vi "Main.vi"(11 "Module Admin":refnum<class "Delacor_lib_QMH_Module Admin.lvclass">) -> ()   [LabVIEW 2023, in "Dispatcher.lvlib"]
doc: "This template is based off of the Queued Message Handler design pattern and the Queued Message Handler project template that ships with LabVIEW.\n\nThe main difference is that the queue is private to this module and communication between modules is performed via Broadcast and Request events.\n\nRequest events are wrapped in public API methods and are handled in the Event Handling Loop (EHL) of this VI. Any module can register for Broadcast events sent by this module. The EHL generates messages based on user interface actions.\n\nThe Message Handling Loop (MHL) processes messages generated by the EHL, or by other messages. The messages are string values, so new messages can be added easily to the Message Cases case structure in the MHL. Each message cluster can also provide an optional value for Message Data, which is a variant that can be converted to whatever message-specific data is required.\n_____\nBased on DQMH Project Template 6.1.0.94."
uses:
  Dispatcher.lvlib
  <vilib>/Delacor/Delacor QMH/Libraries/Message Queue_class/Delacor_lib_QMH_Message Queue.lvclass
  Module Data--cluster.ctl
  <vilib>/Utility/miscctls.llb/LVPointTypeDef.ctl
  <vilib>/Utility/error.llb/Error Cluster From Error Code.vi
  <vilib>/ErrorRing/Error Ring.xnode
  <vilib>/Delacor/Delacor QMH/Libraries/Message Queue_class/Delacor_lib_QMH_Enqueue Message (Single).vi
  Stop Argument--cluster.ctl
  <vilib>/Delacor/Delacor QMH/Libraries/Module Admin_class/Delacor_lib_QMH_Module Admin.lvclass
  Registration/Registration.lvlib
  Graph_data_collector/Graph_data_collector.lvlib
  Initial Data/Initial Data.lvlib
  Registration/Data_reg.ctl
  Graph_data_collector/Data Control.ctl
  <vilib>/Delacor/Delacor QMH/Libraries/Message Queue_class/Delacor_lib_QMH_Enqueue Message (Array).vi
panel:
  out "error out":errorcluster
  # "Загрузка......"
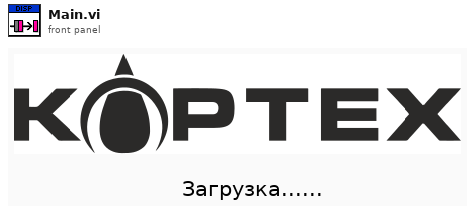
[diagram p1: front panel]
types:
  T1 = typedef "Dispatcher.lvlib/Request Events--cluster.ctl" = cluster{"Stop Module":refnum<user-event>, "Show Panel":refnum<user-event>, "Hide Panel":refnum<user-event>, "Get Module Execution Status":refnum<user-event>, "Show Diagram":refnum<user-event>}
  T2 = typedef "Calculator.lvlib/Broadcast Events--cluster.ctl" = cluster{"Module Did Init":refnum<user-event>, "Status Updated":refnum<user-event>, "Error Reported":refnum<user-event>, "Module Did Stop":refnum<user-event>, "Update Module Execution Status":refnum<user-event>}
  T3 = typedef "Pressure Control System.lvlib/Broadcast Events--cluster.ctl" = cluster{"Module Did Init":refnum<user-event>, "Status Updated":refnum<user-event>, "Error Reported":refnum<user-event>, "Module Did Stop":refnum<user-event>, "Update Module Execution Status":refnum<user-event>}
  T4 = typedef "Automatic.lvlib/Broadcast Events--cluster.ctl" = cluster{"Module Did Init":refnum<user-event>, "Status Updated":refnum<user-event>, "Error Reported":refnum<user-event>, "Module Did Stop":refnum<user-event>, "Update Module Execution Status":refnum<user-event>, "Next Step":refnum<user-event>}
  T5 = typedef "Heat UI.lvlib/Broadcast Events--cluster.ctl" = cluster{"Module Did Init":refnum<user-event>, "Status Updated":refnum<user-event>, "Error Reported":refnum<user-event>, "Module Did Stop":refnum<user-event>, "Update Module Execution Status":refnum<user-event>, "T Data":refnum<user-event>}
  T6 = typedef "DMX.lvlib/Broadcast Events--cluster.ctl" = cluster{"Module Did Init":refnum<user-event>, "Status Updated":refnum<user-event>, "Error Reported":refnum<user-event>, "Module Did Stop":refnum<user-event>, "Update Module Execution Status":refnum<user-event>, "DMX Data":refnum<user-event>}
  T7 = typedef "Initial Data.lvlib/Broadcast Events--cluster.ctl" = cluster{"Module Did Init":refnum<user-event>, "Status Updated":refnum<user-event>, "Error Reported":refnum<user-event>, "Module Did Stop":refnum<user-event>, "Update Module Execution Status":refnum<user-event>, "Data":refnum<user-event>}
  T8 = typedef "LCR GWinstek.lvlib/Broadcast Events--cluster.ctl" = cluster{"Module Did Init":refnum<user-event>, "Status Updated":refnum<user-event>, "Error Reported":refnum<user-event>, "Module Did Stop":refnum<user-event>, "Update Module Execution Status":refnum<user-event>, "LCR Data":refnum<user-event>}
  T9 = typedef "Manual.lvlib/Broadcast Events--cluster.ctl" = cluster{"Module Did Init":refnum<user-event>, "Status Updated":refnum<user-event>, "Error Reported":refnum<user-event>, "Module Did Stop":refnum<user-event>, "Update Module Execution Status":refnum<user-event>, "Pump Data":refnum<user-event>}
  T10 = typedef "Separator UZ.lvlib/Broadcast Events--cluster.ctl" = cluster{"Module Did Init":refnum<user-event>, "Status Updated":refnum<user-event>, "Error Reported":refnum<user-event>, "Module Did Stop":refnum<user-event>, "Update Module Execution Status":refnum<user-event>, "Time Data":refnum<user-event>}
  T11 = typedef "Graph_data_collector.lvlib/Broadcast Events--cluster.ctl" = cluster{"Module Did Init":refnum<user-event>, "Status Updated":refnum<user-event>, "Error Reported":refnum<user-event>, "Module Did Stop":refnum<user-event>, "Update Module Execution Status":refnum<user-event>}
  T12 = typedef "Registration.lvlib/Broadcast Events--cluster.ctl" = cluster{"Module Did Init":refnum<user-event>, "Status Updated":refnum<user-event>, "Error Reported":refnum<user-event>, "Module Did Stop":refnum<user-event>, "Update Module Execution Status":refnum<user-event>, "Data from Registration":refnum<user-event>, "Get Main VI Reference":refnum<user-event>}
  T13 = typedef "Log Module.lvlib/Broadcast Events--cluster.ctl" = cluster{"Module Did Init":refnum<user-event>, "Status Updated":refnum<user-event>, "Error Reported":refnum<user-event>, "Module Did Stop":refnum<user-event>, "Update Module Execution Status":refnum<user-event>}
  T14 = typedef "Menu.lvlib/Broadcast Events--cluster.ctl" = cluster{"Module Did Init":refnum<user-event>, "Status Updated":refnum<user-event>, "Error Reported":refnum<user-event>, "Module Did Stop":refnum<user-event>, "Update Module Execution Status":refnum<user-event>}
  T15 = typedef "Dispatcher.lvlib/Module Data--cluster.ctl" = cluster{"Status":string, "Data reg":T16}
  T16 = typedef "Registration.lvlib/Data_reg.ctl" = cluster{"Дата":string, "Время":string, "Рпл1, МПа":dbl, "Vпл, см3":dbl, "Рпл2, МПа":dbl, "Ргор, МПа":dbl, "Рэфф, МПа":dbl, "R, Ом":dbl, "dL, мм":dbl, "Ткд, градС":dbl, "Тпрод, мкс":dbl, "Тпоп.1, мкс":dbl, "Тпоп.2, мкс":dbl, "Рдм, МПа":dbl, "Q, мл":dbl, "Тнагр, градС":dbl, "ЦАП, градС":dbl}
  T17 = enum32{"invalid lock state", "Not Locked", "Locked (No Password)", "Password-protected"}
  T18 = typedef "Dispatcher.lvlib/Stop Argument--cluster.ctl" = cluster{"Origin":string, "Exit via Stop Module Req?":bool, "Wait for Module to stop?":bool}
  T19 = typedef "LVPointTypeDef.ctl" = cluster{"Horizontal":i16, "Vertical":i16}
  T20 = enum32{"Invalid", "Standard", "Closed", "Hidden", "Minimized", "Maximized"}
  T21 = typedef "Graph_data_collector.lvlib/Data Control.ctl" = cluster{"Время":dbl, "Рпл1, МПа":dbl, "Vпл, см3":dbl, "Рпл2, МПа":dbl, "Ргор, МПа":dbl, "Ткд, градС":dbl, "R, Ом":dbl, "dL, мм":dbl, "Рэфф, МПа":dbl, "Рдм, МПа":dbl, "Q, мл":dbl, "Тнагр, градС":dbl, "ЦАП, градС":dbl}
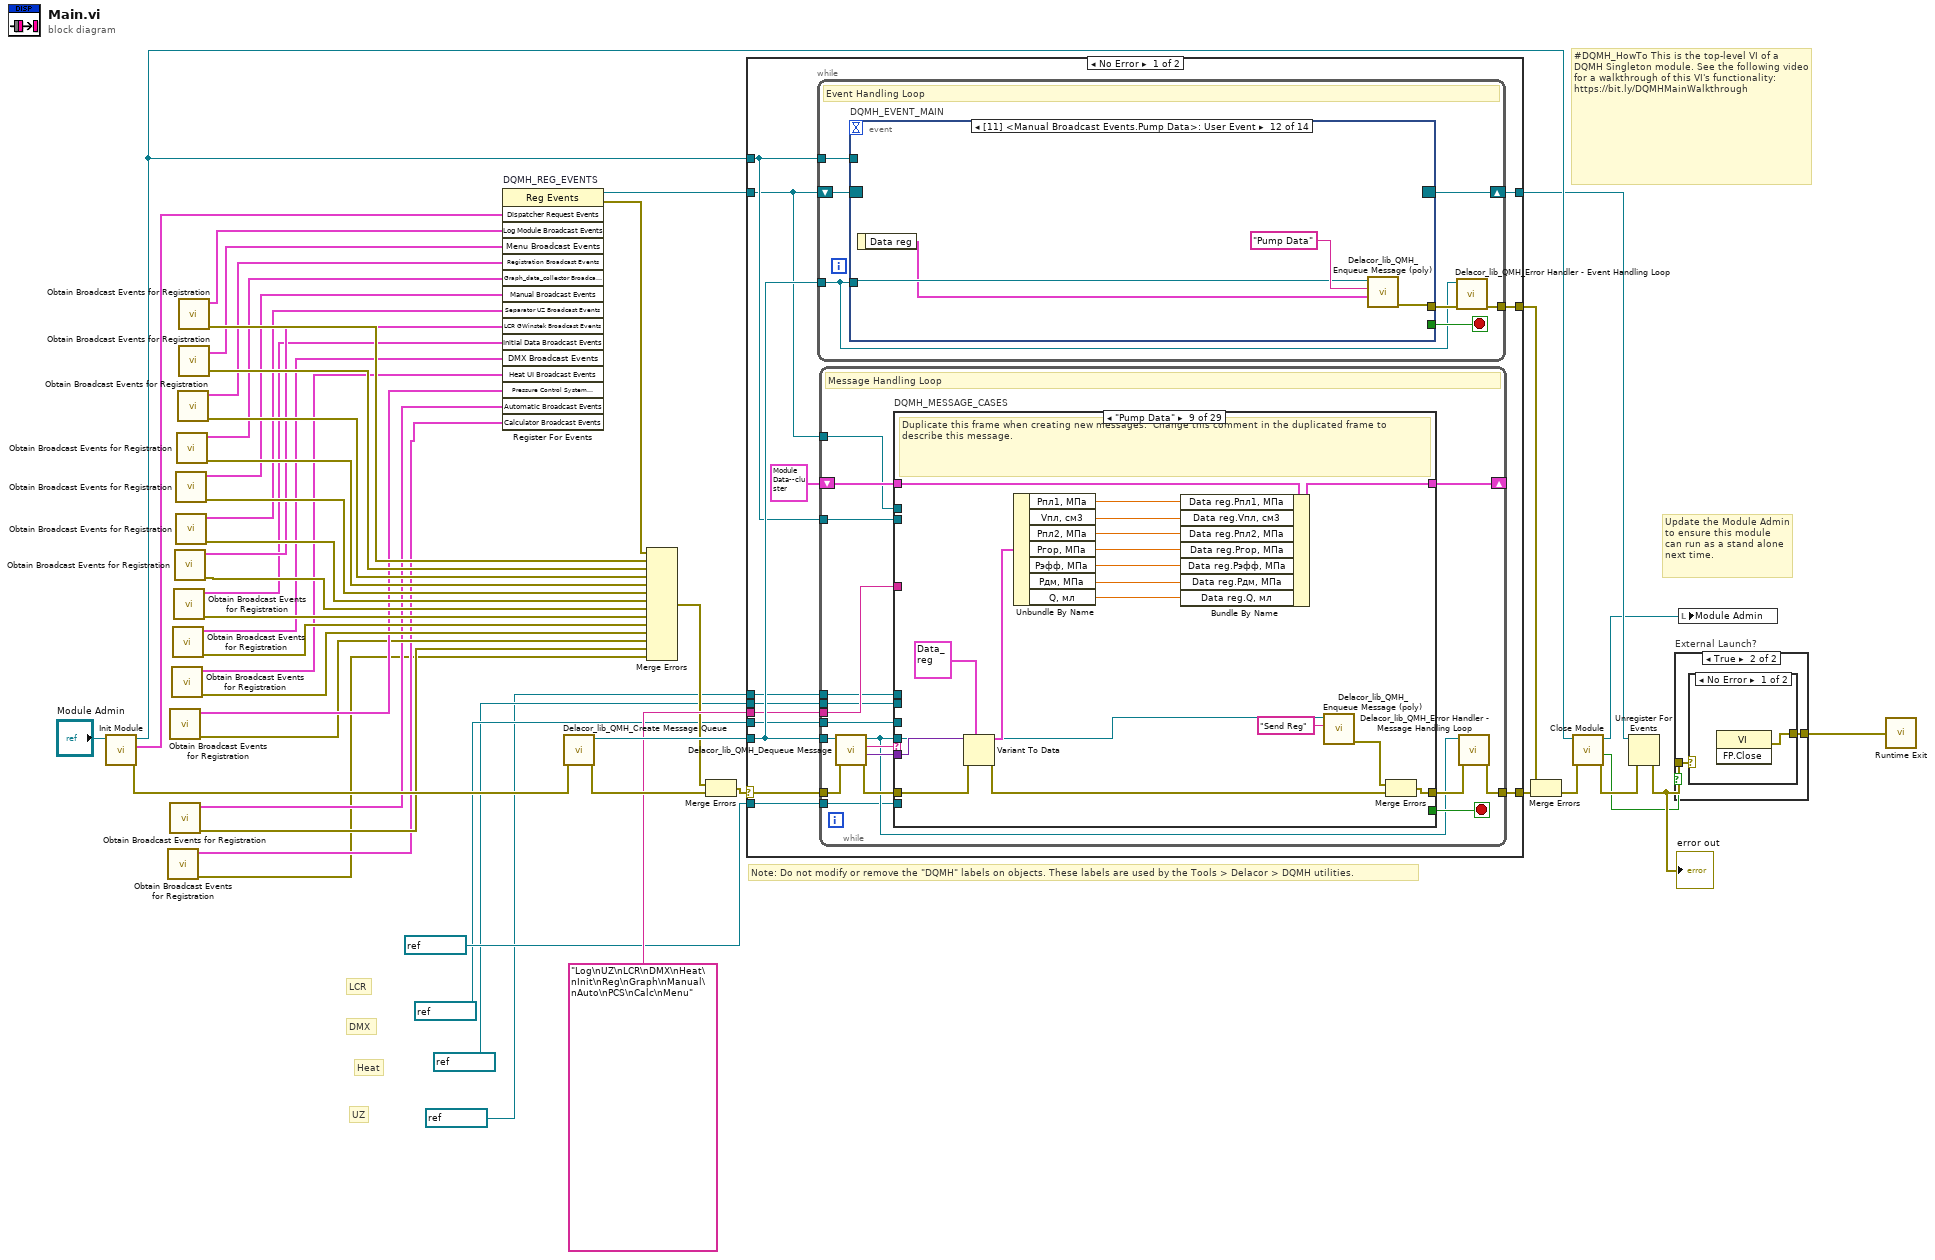
[diagram p0: block diagram]
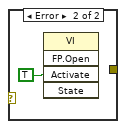
[diagram p3: hidden frame]
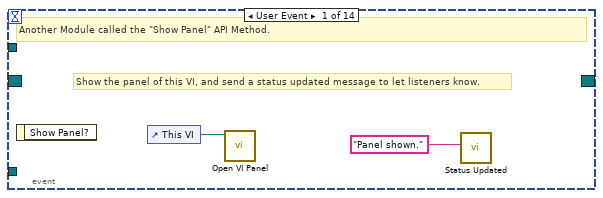
[diagram p4: hidden frame]
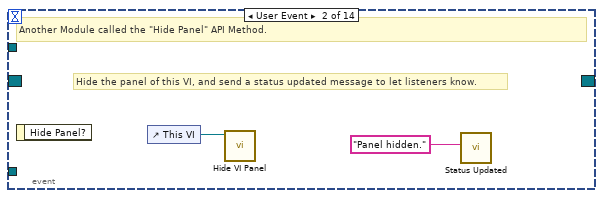
[diagram p5: hidden frame]
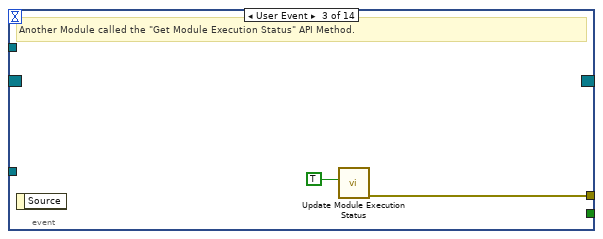
[diagram p6: hidden frame]
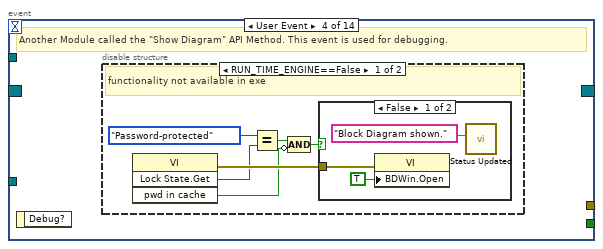
[diagram p7: hidden frame]
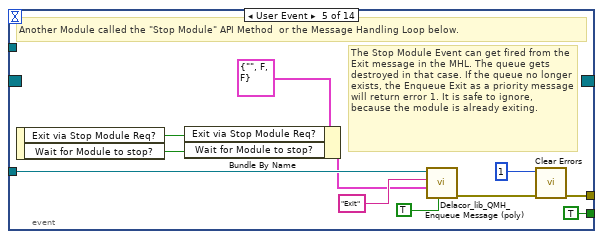
[diagram p10: hidden frame]
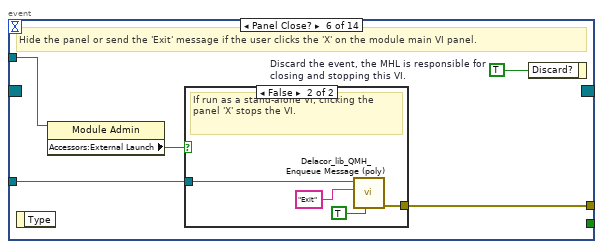
[diagram p11: hidden frame]
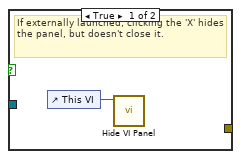
[diagram p12: hidden frame]
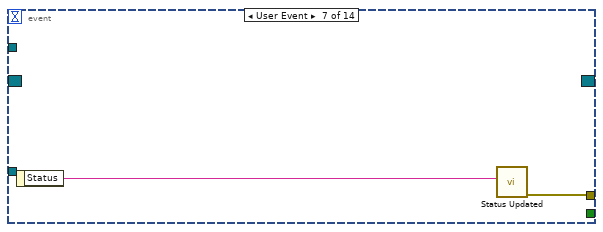
[diagram p13: hidden frame]
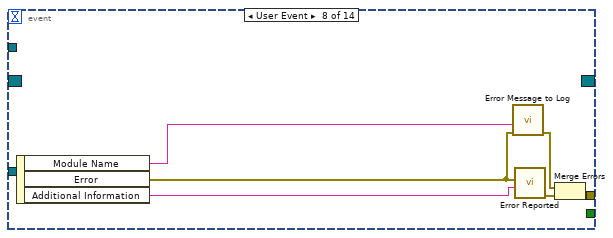
[diagram p14: hidden frame]
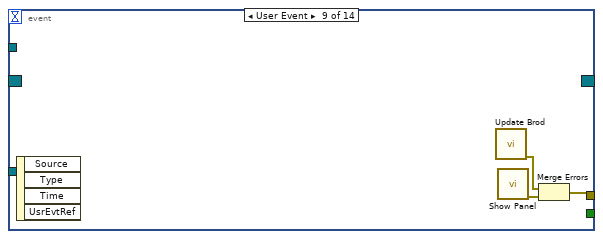
[diagram p15: hidden frame]
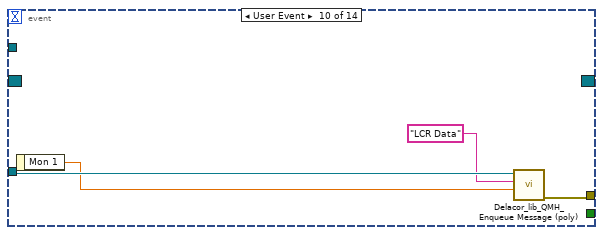
[diagram p16: hidden frame]
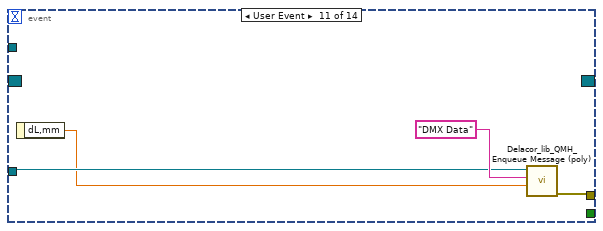
[diagram p17: hidden frame]
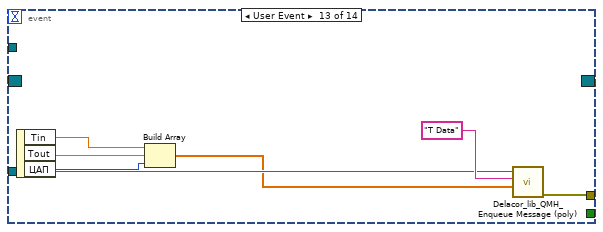
[diagram p18: hidden frame]
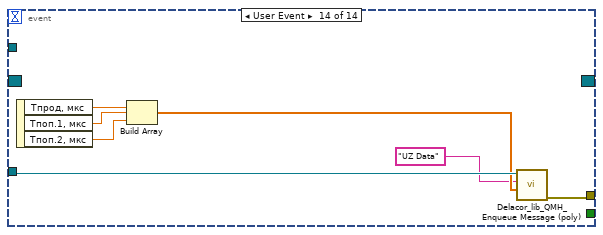
[diagram p19: hidden frame]
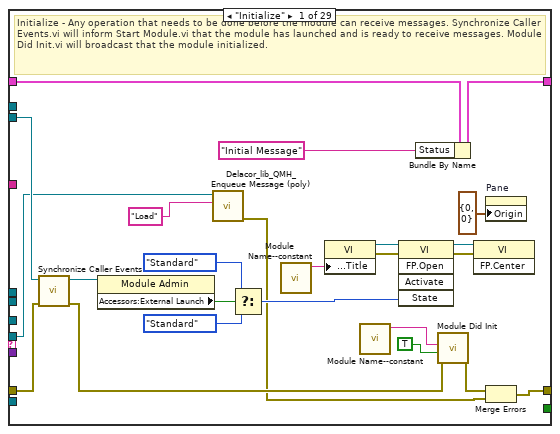
[diagram p20: hidden frame]
diagram:
  # "UZ"
  # "Heat"
  # "DMX"
  # "LCR"
  # "#DQMH_HowTo This is the top-level VI of a DQMH Singleton module. See the following video for a walkthrough of this VI's functionality: https://bit.ly/DQMHMainWalkthrough"
  # "Note: Do not modify or remove the \"DQMH\" labels on objects. These labels are used by the Tools > Delacor > DQMH utilities."
  # "Update the Module Admin to ensure this module can run as a stand alone next time."
  n1 = call "Init Module.vi"("Singleton Module Admin in"="Module Admin") -> ("error out"=w49:errorcluster, "Dispatcher Request Events"=w39:T1, "Singleton Module Admin out"=w42:refnum<class "Delacor_lib_QMH_Module Admin.lvclass">)  [unwired: 8 in]
  n2 = call "Obtain Broadcast Events for Registration.vi"() -> ("error out"=w1:errorcluster, "Calculator Broadcast Events"=w2:T2)  [unwired: 9 in, 1 out]
  n3 = call "Obtain Broadcast Events for Registration.vi"() -> ("error out"=w6:errorcluster, "Pressure Control System Broadcast Events"=w7:T3)  [unwired: 9 in, 1 out]
  n4 = call "Obtain Broadcast Events for Registration.vi"() -> ("error out"=w4:errorcluster, "Automatic Broadcast Events"=w5:T4)  [unwired: 9 in, 1 out]
  n5 = call "Obtain Broadcast Events for Registration.vi"() -> ("error out"=w9:errorcluster, "Heat UI Broadcast Events"=w10:T5)  [unwired: 9 in, 1 out]
  n6 = call "Obtain Broadcast Events for Registration.vi"() -> ("error out"=w12:errorcluster, "DMX Broadcast Events"=w13:T6)  [unwired: 9 in, 1 out]
  n7 = call "Obtain Broadcast Events for Registration.vi"() -> ("error out"=w14:errorcluster, "Initial Data Broadcast Events"=w15:T7)  [unwired: 9 in, 1 out]
  n8 = call "Obtain Broadcast Events for Registration.vi"() -> ("error out"=w17:errorcluster, "LCR GWinstek Broadcast Events"=w18:T8)  [unwired: 9 in, 1 out]
  n9 = call "Obtain Broadcast Events for Registration.vi"() -> ("error out"=w22:errorcluster, "Manual Broadcast Events"=w21:T9)  [unwired: 9 in, 1 out]
  n10 = call "Obtain Broadcast Events for Registration.vi"() -> ("error out"=w19:errorcluster, "Separator UZ Broadcast Events"=w20:T10)  [unwired: 9 in, 1 out]
  n11 = call "Obtain Broadcast Events for Registration.vi"() -> ("error out"=w26:errorcluster, "Graph_data_collector Broadcast Events"=w24:T11)  [unwired: 9 in, 1 out]
  n12 = call "Obtain Broadcast Events for Registration.vi"() -> ("error out"=w27:errorcluster, "Registration Broadcast Events"=w25:T12)  [unwired: 9 in, 1 out]
  n13 = call "Obtain Broadcast Events for Registration.vi"() -> ("error out"=w32:errorcluster, "Log Module Broadcast Events"=w33:T13)  [unwired: 9 in, 1 out]
  n14 = call "Obtain Broadcast Events for Registration.vi"() -> ("error out"=w28:errorcluster, "Menu Broadcast Events"=w29:T14)  [unwired: 9 in, 1 out]
  n15 = register-events "DQMH_REG_EVENTS"(w39, w33, w29, w25, w24, w21, w20, w18, w15, w13, w10, w7, w5, w2) -> (reference out=w40:refnum<event-registration>, error out=w30:errorcluster)  [unwired: 2 in]
  n16 = call <vilib>:"Delacor_lib_QMH_Create Message Queue.vi"("error in"=w49) -> ("error out"=w44:errorcluster, "Message Queue"=w38:refnum<class "Delacor_lib_QMH_Message Queue.lvclass">)  [unwired: 9 in]
  n17 = Merge Errors(w30, w32, w28, w27, w26, w22, w19, w17, w14, w12, w9, w6, w4, w1) -> (w31:errorcluster)
  n18 = Merge Errors(w31, w44) -> (w43:errorcluster)
  n19 = case shown="No Error" w43 {
    selector: w43 -> [w61 w479]
    tunnel: [w63 w478] -> w50
    tunnel: [w60 w484] -> w41
    tunnel: w40 -> [w55 w484]
    tunnel: w38 -> [w58 w477]
    tunnel: [w62 _] -> w47
    tunnel: w42 -> [w57 w480]
    tunnel: "Log\nUZ\nLCR\nDMX\nHeat\nInit\nReg\nGraph\nManual\nAuto\nPCS\nCalc\nMenu" -> [w56 _]
    tunnel: refnum<visa-resource-name> "COM3" ("VISA resource name") -> [w54 _]
    tunnel: refnum<visa-resource-name> "COM2" ("COM") -> [w53 _]
    tunnel: refnum<visa-resource-name> "COM1" ("VISA resource name") -> [w52 _]
    tunnel: refnum<visa-resource-name> "COM4" ("COM") -> [w51 _]
    frame No Error {
      n20 = while {
        tunnel: w58 -> [w64]
        shift-right: [w67] -> w60
        shift-left: w55 -> [w68]
        tunnel: [w69] -> w62
        tunnel: w57 -> [w65]
        stop <- w66 stop-if-true
        # "Event Handling Loop"
        n21 = event "DQMH_EVENT_MAIN" shown="[11] <Manual Broadcast Events.Pump Data>: User Event" {
          selector: w68 -> [_ _ _ _ _ _ _ _ _ _ _ _ _ _]
          dyn-events: [_ _ _ _ _ _ _ _ _ _ _ _ _ _] -> w67
          timeout: _ -> [_ _ _ _ _ _ _ _ _ _ _ _ _ _]
          tunnel: [_ _ _ _ TRUE ("Discard?") _ _ _ _ _ _ _ _ _] -> w66
          tunnel: w64 -> [_ _ _ _ w92 w99 _ _ _ w120 w124 w128 w134 w139]
          tunnel: [_ _ w76 _ w95 w101 w108 w112 w116 w121 w122 w126 w135 w140] -> w70
          tunnel: w65 -> [_ _ _ _ _ w98 _ _ _ _ _ _ _ _]
          event User Event {
            # "Show the panel of this VI, and send a status updated message to let listeners know."
            # "Another Module called the \"Show Panel\" API Method."
            n22 = event-data() -> ()  [unwired: 1 in, 1 out]
            n23 = control-ref of="This VI"() -> (w72:refnum<vi>)
            n24 = call "Open VI Panel.vi"("VI"=w72) -> ()  [unwired: 10 in, 1 out]
            n25 = call "Status Updated.vi"("Status"="Panel shown." ("format string")) -> ()  [unwired: 10 in, 1 out]
          }
          event User Event {
            # "Hide the panel of this VI, and send a status updated message to let listeners know."
            # "Another Module called the \"Hide Panel\" API Method."
            n26 = event-data() -> ()  [unwired: 1 in, 1 out]
            n27 = control-ref of="This VI"() -> (w74:refnum<vi>)
            n28 = call "Hide VI Panel.vi"("VI"=w74) -> ()  [unwired: 10 in, 1 out]
            n29 = call "Status Updated.vi"("Status"="Panel hidden." ("format string")) -> ()  [unwired: 10 in, 1 out]
          }
          event User Event {
            # "Another Module called the \"Get Module Execution Status\" API Method."
            n30 = event-data() -> ()  [unwired: 1 in, 1 out]
            n31 = call "Update Module Execution Status.vi"("Running?"=TRUE) -> ("error out"=w76:errorcluster)  [unwired: 10 in]
          }
          event User Event {
            # "Another Module called the \"Show Diagram\" API Method. This event is used for debugging."
            n32 = event-data() -> ()  [unwired: 1 in, 1 out]
            n33 = disable-structure shown="RUN_TIME_ENGINE==False" {
              frame condition #0 (active) {
                # "functionality not available in exe"
                n34 = invoke class="VI" method="Lock State.Get"() -> (error out=w82:errorcluster, "Get Lock State"=w81:T17, "pwd in cache"=w78:bool)  [unwired: 4 in, 1 out]
                n35 = Equal?(x=T17."Password-protected", y=w81) -> (x = y?=w79:bool)
                n36 = Compound Arithmetic op=AND(w79, invert w78) -> (w77:bool)
                n37 = case shown="False" w77 {
                  tunnel: w82 -> [w85 _]
                  frame False {
                    n38 = property class="VI"(error in=w85, "BDWin.Open"=TRUE ("Block Diagram Window:Open")) -> ()  [unwired: 1 in, 2 out]
                    n39 = call "Status Updated.vi"("Status"="Block Diagram shown." ("format string")) -> ()  [unwired: 10 in, 1 out]
                  }
                  frame True {
                    # "Password-protected VI, and the password is not in the cache. Do not show the diagram."
                  }
                }
              }
              frame condition #1 {
              }
            }
          }
          event User Event {
            # "The Stop Module Event can get fired from the Exit message in the MHL. The queue gets destroyed in that case. If the queue no longer exists, the Enqueue Exit as a priority message will return error 1. It is safe to ignore, because the module is already exiting."
            # "Another Module called the \"Stop Module\" API Method  or the Message Handling Loop below."
            n40 = event-data() -> ("Exit via Stop Module Req?"=w88:bool, "Wait for Module to stop?"=w87:bool)  [unwired: 1 in]
            n41 = Bundle By Name(cluster=T18 {"Origin"="", "Exit via Stop Module Req?"=FALSE, "Wait for Module to stop?"=FALSE} ("Stop Argument"), "Exit via Stop Module Req?"=w88, "Wait for Module to stop?"=w87) -> (w86:T18)
            n42 = call-poly <vilib>:"Delacor_lib_QMH_Enqueue Message (poly).vi"("Priority Message? (F)"=TRUE, "Message Data"=w86, "Message"="Exit", "Message Queue in"=w92) -> ("error out"=w96:errorcluster)  [unwired: 6 in, 1 out]
            n43 = call <vilib>:"Clear Errors.vi"("error in (no error)"=w96, "specific error code to clear (0: all)"=1) -> ("error out"=w95:errorcluster)  [unwired: 4 in, 1 out]
          }
          event Panel Close? {
            w100 = TRUE  # Discard the event, the MHL is responsible for closing and stopping this VI.
            # "Hide the panel or send the 'Exit' message if the user clicks the 'X' on the module main VI panel."
            n44 = event-data() -> ()  [unwired: 1 in, 1 out]
            n45 = property class="Module Admin"(reference=w98) -> ("Accessors:External Launch"=w97:bool)  [unwired: 1 in, 2 out]
            n46 = case shown="False" w97 {
              tunnel: w99 -> [_ w105]
              tunnel: [_ w106] -> w101
              frame True {
                # "If externally launched, clicking the 'X' hides the panel, but doesn't close it."
                n47 = control-ref of="This VI"() -> (w102:refnum<vi>)
                n48 = call "Hide VI Panel.vi"("VI"=w102) -> ()  [unwired: 10 in, 1 out]
              }
              frame False {
                # "If run as a stand-alone VI, clicking the panel 'X' stops the VI."
                n49 = call-poly <vilib>:"Delacor_lib_QMH_Enqueue Message (poly).vi"("Priority Message? (F)"=TRUE, "Message"="Exit", "Message Queue in"=w105) -> ("error out"=w106:errorcluster)  [unwired: 7 in, 1 out]
              }
            }
            n50 = event-data("Discard?"=w100) -> ()  [unwired: 1 in, 1 out]
          }
          event User Event {
            n51 = event-data() -> ("Status"=w107:string)  [unwired: 1 in]
            n52 = call "Status Updated.vi"("Status"=w107) -> ("error out"=w108:errorcluster)  [unwired: 10 in]
          }
          event User Event {
            n53 = event-data() -> ("Module Name"=w109:string, "Error"=w110:errorcluster, "Additional Information"=w113:string)  [unwired: 1 in]
            n54 = call "Error Message to Log.vi"("Error In"=w110, "Source"=w109) -> ("Error Out"=w111:errorcluster)  [unwired: 9 in]
            n55 = call "Error Reported.vi"("Additional Information"=w113, "Error"=w110) -> ("error out"=w114:errorcluster)  [unwired: 9 in]
            n56 = Merge Errors(w111, w114) -> (w112:errorcluster)
          }
          event User Event {
            n57 = event-data() -> ()  [unwired: 1 in, 4 out]
            n58 = call "Update Brod.vi"() -> ("error out"=w115:errorcluster)  [unwired: 11 in]
            n59 = call "Show Panel.vi"() -> ("error out"=w117:errorcluster)  [unwired: 11 in]
            n60 = Merge Errors(w115, w117) -> (w116:errorcluster)
          }
          event User Event {
            n61 = event-data() -> ("Mon 1"=w119:dbl)  [unwired: 1 in]
            n62 = call-poly <vilib>:"Delacor_lib_QMH_Enqueue Message (poly).vi"("Message Data"=w119, "Message"="LCR Data", "Message Queue in"=w120) -> ("error out"=w121:errorcluster)  [unwired: 7 in, 1 out]
          }
          event User Event {
            n63 = event-data() -> ("dL,mm"=w123:dbl)  [unwired: 1 in]
            n64 = call-poly <vilib>:"Delacor_lib_QMH_Enqueue Message (poly).vi"("Message Data"=w123, "Message"="DMX Data", "Message Queue in"=w124) -> ("error out"=w122:errorcluster)  [unwired: 7 in, 1 out]
          }
          event User Event {
            n65 = event-data() -> ("Data reg"=w127:T16)  [unwired: 1 in]
            n66 = call-poly <vilib>:"Delacor_lib_QMH_Enqueue Message (poly).vi"("Message Data"=w127, "Message"="Pump Data", "Message Queue in"=w128) -> ("error out"=w126:errorcluster)  [unwired: 7 in, 1 out]
          }
          event User Event {
            n67 = event-data() -> ("Tin"=w133:dbl, "Tout"=w132:dbl, "ЦАП"=w131:i16)  [unwired: 1 in]
            n68 = Build Array(w133, w132, w131) -> (w130:dbl[])
            n69 = call-poly <vilib>:"Delacor_lib_QMH_Enqueue Message (poly).vi"("Message Data"=w130, "Message"="T Data", "Message Queue in"=w134) -> ("error out"=w135:errorcluster)  [unwired: 7 in, 1 out]
          }
          event User Event {
            n70 = event-data() -> ("Тпрод, мкс"=w143:dbl, "Тпоп.1, мкс"=w142:dbl, "Тпоп.2, мкс"=w141:dbl)  [unwired: 1 in]
            n71 = Build Array(w143, w142, w141) -> (w138:dbl[])
            n72 = call-poly <vilib>:"Delacor_lib_QMH_Enqueue Message (poly).vi"("Message Data"=w138, "Message"="UZ Data", "Message Queue in"=w139) -> ("error out"=w140:errorcluster)  [unwired: 7 in, 1 out]
          }
        }
        n73 = call-dynamic "Delacor_lib_QMH_Error Handler - Event Handling Loop.vi"("error in"=w70, "Message Queue in"=w64) -> ("dup error in"=w69:errorcluster)  [unwired: 8 in, 1 out]
      }
      n74 = while {
        tunnel: w58 -> [w152]
        shift-right: [w156] -> _
        shift-left: T15 {"Status"="", "Data reg"={"Дата"="", "Время"="", "Рпл1, МПа"=0.0, "Vпл, см3"=0.0, "Рпл2, МПа"=0.0, "Ргор, МПа"=0.0, "Рэфф, МПа"=0.0, "R, Ом"=0.0, "dL, мм"=0.0, "Ткд, градС"=0.0, "Тпрод, мкс"=0.0, "Тпоп.1, мкс"=0.0, "Тпоп.2, мкс"=0.0, "Рдм, МПа"=0.0, "Q, мл"=0.0, "Тнагр, градС"=0.0, "ЦАП, градС"=0.0}} ("Data Cluster") -> [w157]
        tunnel: w61 -> [w160]
        tunnel: [w158] -> w63
        tunnel: w57 -> [w150]
        tunnel: w56 -> [w149]
        tunnel: w55 -> [w148]
        tunnel: w54 -> [w147]
        tunnel: w53 -> [w146]
        tunnel: w52 -> [w145]
        tunnel: w51 -> [w144]
        stop <- w155 stop-if-true
        # "Message Handling Loop"
        n75 = call-dynamic "Delacor_lib_QMH_Dequeue Message.vi"("error in"=w160, "Message Queue in"=w152) -> ("error out"=w159:errorcluster, "Message Data"=w153:variant, "Message"=w154:string, "Message Queue out"=w151:refnum<class "Delacor_lib_QMH_Message Queue.lvclass">)  [unwired: 6 in]
        n76 = case "DQMH_MESSAGE_CASES" shown="\"Pump Data\"" w154 {
          selector: w154 -> [_ _ _ _ _ _ _ _ _ _ _ _ _ _ _ _ _ _ _ _ _ _ _ _ _ _ _ _ w464]
          tunnel: w151 -> [w162 _ _ _ _ _ _ _ w253 _ _ _ _ _ _ _ _ _ _ _ _ _ _ w402 _ _ w429 w457 _]
          tunnel: w159 -> [w183 w187 w190 w211 w216 w227 w238 w246 w264 w279 w288 w297 w307 w316 w326 w336 w345 w355 w365 w374 w383 w392 _ w408 w414 w419 w436 w462 w466]
          tunnel: [w165 w187 w189 w210 w219 w230 w241 w249 w267 w278 w287 w296 w306 w315 w325 w335 w344 w354 w364 w373 w382 w391 w396 w407 w414 w418 w432 w459 w467] -> w161
          tunnel: w157 -> [w172 w186 w188 w209 w218 w229 w240 w248 w266 w277 w286 w295 w305 w314 w324 w334 w343 w353 w363 w372 w381 w390 w395 w406 w413 w416 w431 w456 w465]
          tunnel: [w171 w186 w188 w209 w213 w225 w236 w243 w262 w277 w286 w295 w305 w314 w324 w334 w343 w353 w363 w372 w381 w390 w395 w406 w413 w416 w431 w456 w465] -> w156
          tunnel: [_ _ _ _ _ _ _ _ _ _ _ _ _ _ _ _ _ _ _ _ _ _ _ _ _ _ _ w455 _] -> w155
          tunnel: w153 -> [_ _ _ _ w215 w226 w237 w245 w263 _ _ _ _ _ _ _ _ _ _ _ _ _ _ _ _ _ w430 w454 _]
          tunnel: w150 -> [w173 _ _ _ _ _ _ _ _ _ _ _ _ _ _ _ _ _ _ _ _ _ _ _ _ _ w428 w449 _]
          tunnel: w149 -> [_ _ _ _ _ _ _ _ _ _ _ _ _ _ _ _ _ _ _ _ _ _ _ w397 _ _ _ _ _]
          tunnel: w148 -> [_ _ _ _ _ _ _ _ _ w276 w285 w294 w304 w313 w323 w333 w342 w352 w362 w371 w380 w389 _ _ _ _ _ _ _]
          tunnel: w147 -> [_ _ _ _ _ _ _ _ _ _ _ _ _ _ w317 _ _ _ _ _ _ _ _ _ _ _ _ _ _]
          tunnel: w146 -> [_ _ _ _ _ _ _ _ _ _ _ _ _ _ _ _ _ w346 _ _ _ _ _ _ _ _ _ _ _]
          tunnel: w145 -> [_ _ _ _ _ _ _ _ _ _ _ _ _ _ _ w327 _ _ _ _ _ _ _ _ _ _ _ _ _]
          tunnel: w144 -> [_ _ _ _ _ _ _ _ _ _ _ _ _ _ _ _ _ _ w356 _ _ _ _ _ _ _ _ _ _]
          frame "Initialize" {
            # "Initialize - Any operation that needs to be done before the module can receive messages. Synchronize Caller Events.vi will inform Start Module.vi that the module has launched and is ready to receive messages. Module Did Init.vi will broadcast that the module initialized."
            n77 = call "Synchronize Caller Events.vi"("error in (no error)"=w183, "Singleton Module Admin in"=w173) -> ("error out"=w182:errorcluster, "Singleton Module Admin out"=w168:refnum<class "Delacor_lib_QMH_Module Admin.lvclass">)  [unwired: 8 in]
            n78 = property class="Module Admin"(reference=w168) -> ("Accessors:External Launch"=w177:bool)  [unwired: 1 in, 2 out]
            n79 = call-poly <vilib>:"Delacor_lib_QMH_Enqueue Message (poly).vi"("Message"="Load", "Message Queue in"=w162) -> ("error out"=w164:errorcluster)  [unwired: 8 in, 1 out]
            n80 = Select(t=T20."Standard" ("State"), s=w177, f=T20."Standard" ("State")) -> (s? t:f=w174:T20)
            n81 = call "Module Name--constant.vi"() -> ("Module Name"=w180:string)  [unwired: 11 in]
            n82 = property class="VI"("Front Panel.Title"=w180) -> (reference out=w179:refnum<vi>, error out=w185:errorcluster)  [unwired: 2 in]
            n83 = call "Module Name--constant.vi"() -> ("Module Name"=w169:string)  [unwired: 11 in]
            n84 = invoke class="VI" method="FP.Open"(reference=w179, error in=w185, "State"=w174) -> (reference out=w178:refnum<vi>, error out=w184:errorcluster)  [unwired: 2 in, 3 out]
            n85 = Bundle By Name(cluster=w172, "Status"="Initial Message" ("Initial Message")) -> (w171:T15)
            n86 = call "Module Did Init.vi"("error in (no error)"=w182, "Initialized?"=TRUE, "Origin"=w169) -> ("error out"=w181:errorcluster)  [unwired: 8 in]
            n87 = invoke class="VI" method="FP.Center"(reference=w178, error in=w184) -> ()  [unwired: 1 in, 3 out]
            n88 = property on="Pane" class="Pane"("Origin"=T19 {"Horizontal"=0, "Vertical"=0}) -> ()  [unwired: 2 in, 2 out]
            n89 = Merge Errors(w181, w164) -> (w165:errorcluster)
          }
          frame "---Module Specific---" {
            # "Separator -- The following cases handle messages specific to this Module."
          }
          frame "---Copy This Frame---" {
            # "Duplicate this frame when creating new messages.  Change this comment in the duplicated frame to describe this message."
            n90 = Merge Errors(w190) -> (w189:errorcluster)
          }
          frame "Send Reg" {
            # "Duplicate this frame when creating new messages.  Change this comment in the duplicated frame to describe this message."
            n91 = Unbundle By Name(w209) -> ("Data reg"=w196:T16, "Data reg.Рпл1, МПа"=w205:dbl, "Data reg.Vпл, см3"=w204:dbl, "Data reg.Рпл2, МПа"=w203:dbl, "Data reg.Ргор, МПа"=w202:dbl, "Data reg.Рэфф, МПа"=w201:dbl, "Data reg.R, Ом"=w200:dbl, "Data reg.dL, мм"=w199:dbl, "Data reg.Ткд, градС"=w198:dbl, "Data reg.Рдм, МПа"=w194:dbl, "Data reg.Q, мл"=w193:dbl, "Data reg.Тнагр, градС"=w192:dbl, "Data reg.ЦАП, градС"=w191:dbl)
            n92 = Bundle By Name(cluster=T21 {"Время"=0.0, "Рпл1, МПа"=0.0, "Vпл, см3"=0.0, "Рпл2, МПа"=0.0, "Ргор, МПа"=0.0, "Ткд, градС"=0.0, "R, Ом"=0.0, "dL, мм"=0.0, "Рэфф, МПа"=0.0, "Рдм, МПа"=0.0, "Q, мл"=0.0, "Тнагр, градС"=0.0, "ЦАП, градС"=0.0} ("Data"), "Рпл1, МПа"=w205, "Vпл, см3"=w204, "Рпл2, МПа"=w203, "Ргор, МПа"=w202, "Рэфф, МПа"=w201, "R, Ом"=w200, "dL, мм"=w199, "Ткд, градС"=w198, "Рдм, МПа"=w194, "Q, мл"=w193, "Тнагр, градС"=w192, "ЦАП, градС"=w191) -> (w197:T21)
            n93 = call "Mes Data.vi"("Data reg"=w196) -> ("error out"=w195:errorcluster)  [unwired: 10 in]
            n94 = call "New_Data.vi"("Data reg"=w196) -> ("error out"=w208:errorcluster)  [unwired: 10 in]
            n95 = call "New_Data.vi"("Graph_Data"=w197) -> ("error out"=w207:errorcluster)  [unwired: 10 in]
            n96 = Merge Errors(w195, w207, w208, w211) -> (w210:errorcluster)
          }
          frame "LCR Data" {
            # "Duplicate this frame when creating new messages.  Change this comment in the duplicated frame to describe this message."
            n97 = Variant To Data(error in=w216, type=0.0 ("Mon 1"), Variant=w215) -> (data=w212:dbl, error out=w217:errorcluster)
            n98 = Bundle By Name(cluster=w218, "Data reg.R, Ом"=w212) -> (w213:T15)
            n99 = Merge Errors(w217) -> (w219:errorcluster)
          }
          frame "UZ Data" {
            # "Duplicate this frame when creating new messages.  Change this comment in the duplicated frame to describe this message."
            n100 = Variant To Data(error in=w227, type=dbl[] [] ("appended array"), Variant=w226) -> (data=w223:dbl[], error out=w228:errorcluster)
            n101 = Index Array(array=w223) -> (element #1=w222:dbl, element #2=w221:dbl, element #3=w220:dbl)  [unwired: 3 in]
            n102 = Bundle By Name(cluster=w229, "Data reg.Тпрод, мкс"=w222, "Data reg.Тпоп.1, мкс"=w221, "Data reg.Тпоп.2, мкс"=w220) -> (w225:T15)
            n103 = Merge Errors(w228) -> (w230:errorcluster)
          }
          frame "T Data" {
            # "Duplicate this frame when creating new messages.  Change this comment in the duplicated frame to describe this message."
            n104 = Variant To Data(error in=w238, type=dbl[] [] ("appended array"), Variant=w237) -> (data=w234:dbl[], error out=w239:errorcluster)
            n105 = Index Array(array=w234) -> (element #1=w233:dbl, element #2=w232:dbl, element #3=w231:dbl)  [unwired: 3 in]
            n106 = Bundle By Name(cluster=w240, "Data reg.Ткд, градС"=w233, "Data reg.Тнагр, градС"=w232, "Data reg.ЦАП, градС"=w231) -> (w236:T15)
            n107 = Merge Errors(w239) -> (w241:errorcluster)
          }
          frame "DMX Data" {
            # "Duplicate this frame when creating new messages.  Change this comment in the duplicated frame to describe this message."
            n108 = Variant To Data(error in=w246, type=0.0 ("Mon 1"), Variant=w245) -> (data=w242:dbl, error out=w247:errorcluster)
            n109 = Bundle By Name(cluster=w248, "Data reg.dL, мм"=w242) -> (w243:T15)
            n110 = Merge Errors(w247) -> (w249:errorcluster)
          }
          frame "Pump Data" {
            # "Duplicate this frame when creating new messages.  Change this comment in the duplicated frame to describe this message."
            n111 = Variant To Data(error in=w264, type=T16 {"Дата"="", "Время"="", "Рпл1, МПа"=0.0, "Vпл, см3"=0.0, "Рпл2, МПа"=0.0, "Ргор, МПа"=0.0, "Рэфф, МПа"=0.0, "R, Ом"=0.0, "dL, мм"=0.0, "Ткд, градС"=0.0, "Тпрод, мкс"=0.0, "Тпоп.1, мкс"=0.0, "Тпоп.2, мкс"=0.0, "Рдм, МПа"=0.0, "Q, мл"=0.0, "Тнагр, градС"=0.0, "ЦАП, градС"=0.0} ("Data reg"), Variant=w263) -> (data=w260:T16, error out=w265:errorcluster)
            n112 = Unbundle By Name(w260) -> ("Рпл1, МПа"=w259:dbl, "Vпл, см3"=w255:dbl, "Рпл2, МПа"=w256:dbl, "Ргор, МПа"=w257:dbl, "Рэфф, МПа"=w258:dbl, "Рдм, МПа"=w251:dbl, "Q, мл"=w250:dbl)
            n113 = Bundle By Name(cluster=w266, "Data reg.Рпл1, МПа"=w259, "Data reg.Vпл, см3"=w255, "Data reg.Рпл2, МПа"=w256, "Data reg.Ргор, МПа"=w257, "Data reg.Рэфф, МПа"=w258, "Data reg.Рдм, МПа"=w251, "Data reg.Q, мл"=w250) -> (w262:T15)
            n114 = call-poly <vilib>:"Delacor_lib_QMH_Enqueue Message (poly).vi"("Message"="Send Reg", "Message Queue in"=w253) -> ("error out"=w254:errorcluster)  [unwired: 8 in, 1 out]
            n115 = Merge Errors(w254, w265) -> (w267:errorcluster)
          }
          frame "Log" {
            # "Duplicate this frame when creating new messages.  Change this comment in the duplicated frame to describe this message."
            n116 = call "Start Module.vi"("Max Logs Allowed"=u32 30, "Log Folder Name"="Logs", "Log Name"="SMP-PS") -> ("error out"=w270:errorcluster, "Wait for Event Sync?"=w272:bool, "Log Module Broadcast Events"=w273:T13)  [unwired: 5 in, 1 out]
            n117 = register-events "DQMH_REG_EVENTS_LOAD"(reference=w276, error in=w270, w273) -> (error out=w271:errorcluster)  [unwired: 13 in, 1 out]
            n118 = call "Synchronize Module Events.vi"("error in (no error)"=w271, "Wait for Event Sync?"=w272) -> ("error out"=w269:errorcluster)  [unwired: 9 in]
            n119 = Merge Errors(w269, w279) -> (w278:errorcluster)
          }
          frame "Menu" {
            # "Duplicate this frame when creating new messages.  Change this comment in the duplicated frame to describe this message."
            n120 = call "Start Module.vi"() -> ("error out"=w284:errorcluster, "Wait for Event Sync?"=w281:bool, "Menu Broadcast Events"=w283:T14)  [unwired: 8 in, 1 out]
            n121 = register-events "DQMH_REG_EVENTS_LOAD"(reference=w285, error in=w284, w283) -> (error out=w282:errorcluster)  [unwired: 13 in, 1 out]
            n122 = call "Synchronize Module Events.vi"("error in"=w282, "Wait for Event Sync?"=w281) -> ("error out"=w280:errorcluster)  [unwired: 9 in]
            n123 = Merge Errors(w280, w288) -> (w287:errorcluster)
          }
          frame "Reg" {
            # "Duplicate this frame when creating new messages.  Change this comment in the duplicated frame to describe this message."
            n124 = call "Start Module.vi"() -> ("error out"=w292:errorcluster, "Wait for Event Sync?"=w291:bool, "Registration Broadcast Events"=w293:T12)  [unwired: 8 in, 1 out]
            n125 = register-events "DQMH_REG_EVENTS_LOAD"(reference=w294, error in=w292, w293) -> (error out=w290:errorcluster)  [unwired: 13 in, 1 out]
            n126 = call "Synchronize Module Events.vi"("error in"=w290, "Wait for Event Sync?"=w291) -> ("error out"=w289:errorcluster)  [unwired: 9 in]
            n127 = Merge Errors(w289, w297) -> (w296:errorcluster)
          }
          frame "Auto" {
            # "Duplicate this frame when creating new messages.  Change this comment in the duplicated frame to describe this message."
            n128 = call "Start Module.vi"() -> ("error out"=w300:errorcluster, "Wait for Event Sync?"=w303:bool, "Automatic Broadcast Events"=w301:T4, "Module ID"=w302:i32)  [unwired: 8 in]
            n129 = register-events "DQMH_REG_EVENTS_LOAD"(reference=w304, error in=w300, w301) -> (error out=w299:errorcluster)  [unwired: 13 in, 1 out]
            n130 = call "Synchronize Module Events.vi"("error in"=w299, "Wait for Event Sync?"=w303, "Module ID in"=w302) -> ("error out"=w298:errorcluster)  [unwired: 7 in, 1 out]
            n131 = Merge Errors(w298, w307) -> (w306:errorcluster)
          }
          frame "Init" {
            # "Duplicate this frame when creating new messages.  Change this comment in the duplicated frame to describe this message."
            n132 = call "Start Module.vi"() -> ("error out"=w310:errorcluster, "Wait for Event Sync?"=w311:bool, "Initial Data Broadcast Events"=w312:T7)  [unwired: 8 in, 1 out]
            n133 = register-events "DQMH_REG_EVENTS_LOAD"(reference=w313, error in=w310, w312) -> (error out=w309:errorcluster)  [unwired: 13 in, 1 out]
            n134 = call "Synchronize Module Events.vi"("error in"=w309, "Wait for Event Sync?"=w311) -> ("error out"=w308:errorcluster)  [unwired: 9 in]
            n135 = Merge Errors(w308, w316) -> (w315:errorcluster)
          }
          frame "LCR" {
            # "Duplicate this frame when creating new messages.  Change this comment in the duplicated frame to describe this message."
            n136 = call "Start Module.vi"("VISA resource name"=w317) -> ("error out"=w320:errorcluster, "Wait for Event Sync?"=w321:bool, "LCR GWinstek Broadcast Events"=w318:T8)  [unwired: 7 in, 1 out]
            n137 = register-events "DQMH_REG_EVENTS_LOAD"(reference=w323, error in=w320, w318) -> (error out=w319:errorcluster)  [unwired: 13 in, 1 out]
            n138 = call "Synchronize Module Events.vi"("error in"=w319, "Wait for Event Sync?"=w321) -> ("error out"=w322:errorcluster)  [unwired: 9 in]
            n139 = Merge Errors(w322, w326) -> (w325:errorcluster)
          }
          frame "Heat" {
            # "Duplicate this frame when creating new messages.  Change this comment in the duplicated frame to describe this message."
            n140 = call "Start Module.vi"("VISA resource name"=w327) -> ("error out"=w331:errorcluster, "Wait for Event Sync?"=w330:bool, "Heat UI Broadcast Events"=w332:T5)  [unwired: 7 in, 1 out]
            n141 = register-events "DQMH_REG_EVENTS_LOAD"(reference=w333, error in=w331, w332) -> (error out=w329:errorcluster)  [unwired: 13 in, 1 out]
            n142 = call "Synchronize Module Events.vi"("error in"=w329, "Wait for Event Sync?"=w330) -> ("error out"=w328:errorcluster)  [unwired: 9 in]
            n143 = Merge Errors(w328, w336) -> (w335:errorcluster)
          }
          frame "PCS" {
            # "Duplicate this frame when creating new messages.  Change this comment in the duplicated frame to describe this message."
            n144 = call "Start Module.vi"() -> ("error out"=w340:errorcluster, "Wait for Event Sync?"=w339:bool, "Pressure Control System Broadcast Events"=w341:T3)  [unwired: 8 in, 1 out]
            n145 = register-events "DQMH_REG_EVENTS_LOAD"(reference=w342, error in=w340, w341) -> (error out=w338:errorcluster)  [unwired: 13 in, 1 out]
            n146 = call "Synchronize Module Events.vi"("error in"=w338, "Wait for Event Sync?"=w339) -> ("error out"=w337:errorcluster)  [unwired: 9 in]
            n147 = Merge Errors(w337, w345) -> (w344:errorcluster)
          }
          frame "DMX" {
            # "Duplicate this frame when creating new messages.  Change this comment in the duplicated frame to describe this message."
            n148 = call "Start Module.vi"("COM"=w346) -> ("error out"=w350:errorcluster, "Wait for Event Sync?"=w349:bool, "DMX Broadcast Events"=w351:T6)  [unwired: 7 in, 1 out]
            n149 = register-events "DQMH_REG_EVENTS_LOAD"(reference=w352, error in=w350, w351) -> (error out=w347:errorcluster)  [unwired: 13 in, 1 out]
            n150 = call "Synchronize Module Events.vi"("error in"=w347, "Wait for Event Sync?"=w349) -> ("error out"=w348:errorcluster)  [unwired: 9 in]
            n151 = Merge Errors(w348, w355) -> (w354:errorcluster)
          }
          frame "UZ" {
            # "Duplicate this frame when creating new messages.  Change this comment in the duplicated frame to describe this message."
            n152 = call "Start Module.vi"("COM"=w356) -> ("error out"=w357:errorcluster, "Wait for Event Sync?"=w361:bool, "Separator UZ Broadcast Events"=w360:T10)  [unwired: 7 in, 1 out]
            n153 = register-events "DQMH_REG_EVENTS_LOAD"(reference=w362, error in=w357, w360) -> (error out=w358:errorcluster)  [unwired: 13 in, 1 out]
            n154 = call "Synchronize Module Events.vi"("error in"=w358, "Wait for Event Sync?"=w361) -> ("error out"=w359:errorcluster)  [unwired: 9 in]
            n155 = Merge Errors(w359, w365) -> (w364:errorcluster)
          }
          frame "Calc" {
            # "Duplicate this frame when creating new messages.  Change this comment in the duplicated frame to describe this message."
            n156 = call "Start Module.vi"() -> ("error out"=w369:errorcluster, "Wait for Event Sync?"=w368:bool, "Calculator Broadcast Events"=w370:T2)  [unwired: 8 in, 1 out]
            n157 = register-events "DQMH_REG_EVENTS_LOAD"(reference=w371, error in=w369, w370) -> (error out=w367:errorcluster)  [unwired: 13 in, 1 out]
            n158 = call "Synchronize Module Events.vi"("error in"=w367, "Wait for Event Sync?"=w368) -> ("error out"=w366:errorcluster)  [unwired: 9 in]
            n159 = Merge Errors(w366, w374) -> (w373:errorcluster)
          }
          frame "Manual" {
            # "Duplicate this frame when creating new messages.  Change this comment in the duplicated frame to describe this message."
            n160 = call "Start Module.vi"() -> ("error out"=w376:errorcluster, "Wait for Event Sync?"=w379:bool, "Manual Broadcast Events"=w377:T9)  [unwired: 8 in, 1 out]
            n161 = register-events "DQMH_REG_EVENTS_LOAD"(reference=w380, error in=w376, w377) -> (error out=w378:errorcluster)  [unwired: 13 in, 1 out]
            n162 = call "Synchronize Module Events.vi"("error in"=w378, "Wait for Event Sync?"=w379) -> ("error out"=w375:errorcluster)  [unwired: 9 in]
            n163 = Merge Errors(w375, w383) -> (w382:errorcluster)
          }
          frame "Graph" {
            # "Duplicate this frame when creating new messages.  Change this comment in the duplicated frame to describe this message."
            n164 = call "Start Module.vi"() -> ("error out"=w387:errorcluster, "Wait for Event Sync?"=w386:bool, "Graph_data_collector Broadcast Events"=w388:T11)  [unwired: 8 in, 1 out]
            n165 = register-events "DQMH_REG_EVENTS_LOAD"(reference=w389, error in=w387, w388) -> (error out=w384:errorcluster)  [unwired: 13 in, 1 out]
            n166 = call "Synchronize Module Events.vi"("error in"=w384, "Wait for Event Sync?"=w386) -> ("error out"=w385:errorcluster)  [unwired: 9 in]
            n167 = Merge Errors(w385, w392) -> (w391:errorcluster)
          }
          frame "Hide" {
            # "Duplicate this frame when creating new messages.  Change this comment in the duplicated frame to describe this message."
            n168 = invoke class="VI" method="FP.Open"("State"=T20."Hidden") -> (error out=w393:errorcluster)  [unwired: 4 in, 4 out]
            n169 = Merge Errors(w393) -> (w396:errorcluster)
          }
          frame "Load" {
            w404 = "%s" ("format string")
            # "Duplicate this frame when creating new messages.  Change this comment in the duplicated frame to describe this message."
            n170 = Spreadsheet String To Array(delimiter (Tab)="\r", format string=w404, spreadsheet string=w397, array type (2D Dbl)=w404) -> (array=w403:string[][])
            n171 = for {
              tunnel: [w412] -> w400
              tunnel: w403 -> [w411] mode=indexing
              tunnel: w402 -> [w410]
              tunnel: [w409] -> w401
              n172 = call-poly <vilib>:"Delacor_lib_QMH_Enqueue Message (poly).vi"("Message Array"=w411, "Message Queue in"=w410) -> ("error out"=w412:errorcluster, "Message Queue out"=w409:refnum<class "Delacor_lib_QMH_Message Queue.lvclass">)  [unwired: 8 in]
            }
            n173 = call-poly <vilib>:"Delacor_lib_QMH_Enqueue Message (poly).vi"("error in"=w400, "Message"="Hide", "Message Queue in"=w401) -> ("error out"=w399:errorcluster)  [unwired: 7 in, 1 out]
            n174 = Merge Errors(w399, w408) -> (w407:errorcluster)
          }
          frame "---Exit and Error Handling---" {
            # "Separator - The following cases handle errors and exit messages."
          }
          frame "Simulate MHL Error" {
            # "#DQMH_HowTo The 'Simulate MHL Error' button  illustrates how the MHL handles errors. This event is instructional in nature and can be removed."
            # "Simulate an error occurring at the MHL"
            n175 = call "Module Name--constant.vi"() -> ("Module Name"=w415:string)  [unwired: 11 in]
            n176 = xnode "Error Ring"("parameter 0"=w415) -> ("error out"=w417:errorcluster)
            n177 = Merge Errors(w419, w417) -> (w418:errorcluster)
          }
          frame "Error" {
            # "#CodeRecommended - If you ever change the name of this \"Error\" message, you'll need to update the name in the Check Loop Error.vi as well."
            # "#CodeRecommended - If the module is running in standalone mode (External Launch = FALSE), this code will pop up an error dialog and call the 'Exit' message if an error occurs. Add more fine-grained error handling here."
            # "Error - Check the error message data and respond accordingly. This message is sent by the \"Error Handler\" VIs at the end of each loop in this application."
            n178 = property class="Module Admin"(reference=w428) -> ("Accessors:External Launch"=w427:bool)  [unwired: 1 in, 2 out]
            n179 = Variant To Data(error in=w436, type=errorcluster {"status"=FALSE, "code"=0, "source"=""} ("error constant"), Variant=w430) -> (data=w437:errorcluster, error out=w434:errorcluster)
            n180 = call "Error Reported.vi"("Error"=w437) -> ()  [unwired: 10 in, 1 out]
            n181 = case shown="False" w427 {
              tunnel: [w442 _] -> w433
              tunnel: w429 -> [w440 _]
              tunnel: w437 -> [w441 _]
              frame False {
                # "If the module is running standalone, then pop up an error dialog and call the \"Exit\" message."
                n182 = call <vilib>:"Simple Error Handler.vi"("error in (no error)"=w441) -> ()  [unwired: 4 in, 5 out]
                n183 = call-poly <vilib>:"Delacor_lib_QMH_Enqueue Message (poly).vi"("Priority Message? (F)"=TRUE, "Message"="Exit", "Message Queue in"=w440) -> ("error out"=w442:errorcluster)  [unwired: 7 in, 1 out]
              }
              frame True {
                # "If the module was launched externally, calling the Error Reported broadcast VI is the only action performed by the \"Error\" message. The module's caller can then process the error appropriately."
              }
            }
            n184 = Merge Errors(w434, w433) -> (w432:errorcluster)
            n185 = local write "error out"(w432) -> ()
          }
          frame "Exit" {
            w453 = 91  # 91: not all Exit messages will have an argument
            w455 = TRUE  # Stop the VI
            # "Release the message queue reference"
            # "Exit - Exit the application."
            n186 = control-ref of="This VI"() -> (w450:refnum<vi>)
            n187 = Variant To Data(error in=w462, type=T18 {"Origin"="", "Exit via Stop Module Req?"=FALSE, "Wait for Module to stop?"=FALSE} ("Stop Argument"), Variant=w454) -> (data=w451:T18, error out=w458:errorcluster)
            n188 = call "Handle Exit.vi"("Stop Argument"=w451, "Admin in"=w449, "VI reference"=w450) -> ("error out"=w448:errorcluster)  [unwired: 7 in, 1 out]
            n189 = call <vilib>:"Clear Errors.vi"("error in (no error)"=w458, "specific error code to clear (0: all)"=w453) -> ("error out"=w461:errorcluster)  [unwired: 4 in, 1 out]
            n190 = call "Stop ext modules.vi"() -> ("error out"=w446:errorcluster)  [unwired: 11 in]
            n191 = call-dynamic "Delacor_lib_QMH_Release Message Queue.vi"("error in"=w461, "Message Queue"=w457) -> ("error out"=w460:errorcluster)  [unwired: 9 in]
            n192 = call <vilib>:"Clear Errors.vi"("error in (no error)"=w446) -> ("error out"=w447:errorcluster)  [unwired: 5 in, 1 out]
            n193 = call "Stop Module.vi"("error in (no error)"=w447, "Wait for Module to Stop? (F)"=TRUE, "Origin"="Exit") -> ("error out"=w445:errorcluster)  [unwired: 8 in]
            n194 = Merge Errors(w445, w446, w448, w460) -> (w459:errorcluster)
          }
          frame Default {
            # "'Default' case only runs if there is a message that isn't defined in any of the other cases.  Output a programming error."
            n195 = call "Module Name--constant.vi"() -> ("Module Name"=w463:string)  [unwired: 11 in]
            n196 = xnode "Error Ring"("parameter 0"=w464, "parameter 1"=w463) -> ("error out"=w468:errorcluster)
            n197 = Merge Errors(w466, w468) -> (w467:errorcluster)
          }
        }
        n198 = call-dynamic "Delacor_lib_QMH_Error Handler - Message Handling Loop.vi"("error in"=w161, "Message Queue in"=w151) -> ("dup error in"=w158:errorcluster)  [unwired: 8 in, 1 out]
      }
    }
    frame Error {
      # "Synchronize Caller Events.vi will inform Start Module.vi that the module has launched and will let the code calling Start Module.vi register for broadcasts and would permit the caller receive the broadcast that an error occurred at launch time."
      n199 = call-dynamic "Delacor_lib_QMH_Release Message Queue.vi"("error in"=w479, "Message Queue"=w477) -> ("error out"=w478:errorcluster)  [unwired: 9 in]
      n200 = call "Synchronize Caller Events.vi"("Singleton Module Admin in"=w480) -> ("error out"=w485:errorcluster)  [unwired: 9 in, 1 out]
      n201 = call "Module Name--constant.vi"() -> ("Module Name"=w483:string)  [unwired: 11 in]
      n202 = Format Into String(format string="An error occurred during initialization. %s is no longer running.", w483) -> (resulting string=w481:string)  [unwired: 2 in, 1 out]
      n203 = Merge Errors(w478, w485) -> (w486:errorcluster)
      n204 = call "Error Reported.vi"("Additional Information"=w481, "Error"=w486) -> ()  [unwired: 9 in, 1 out]
    }
  }
  n205 = Merge Errors(w47, w50) -> (w46:errorcluster)
  n206 = call "Close Module.vi"("error in (no error)"=w46, "Module Admin in"=w42) -> ("error out"=w48:errorcluster, "External Launch"=w35:bool, "Module Admin out"=w36:refnum<class "Delacor_lib_QMH_Module Admin.lvclass">)  [unwired: 7 in]
  n207 = Unregister For Events(event registration refnum=w41, error in=w48) -> (error out=w45:errorcluster)
  "error out" <- w45
  n208 = case "External Launch?" shown="True" w35 {
    tunnel: w45 -> [_ w488]
    tunnel: [_ w487] -> w23
    frame False {
    }
    frame True {
      n209 = case shown="No Error" w488 {
        tunnel: [w489 _] -> w487
        frame No Error {
          n210 = invoke class="VI" method="FP.Close"() -> (error out=w489:errorcluster)  [unwired: 3 in, 2 out]
        }
        frame Error {
          n211 = invoke class="VI" method="FP.Open"("Activate"=TRUE ("Activate?")) -> ()  [unwired: 4 in, 5 out]
        }
      }
    }
  }
  n212 = local write "Module Admin"(w36) -> ()
  n213 = call "Runtime Exit.vi"("error in (no error)"=w23) -> ()
